vi "HTML_GetAllDepFromUsedPlugins.vi"(7 "Framwork Type":T1, 8 "Error In":errorcluster) -> (0 "Error Out":errorcluster, 1 "rel. Filepaths .js":path[](array[path]), 2 "rel. Filepaths .css":path[](array[path]))   [LabVIEW 2014]
uses:
  controls/StylingFrameworks_Enum.ctl
panel:
  # "Private:\nHTML_GetAllDepFromUsedPlugins.vi"
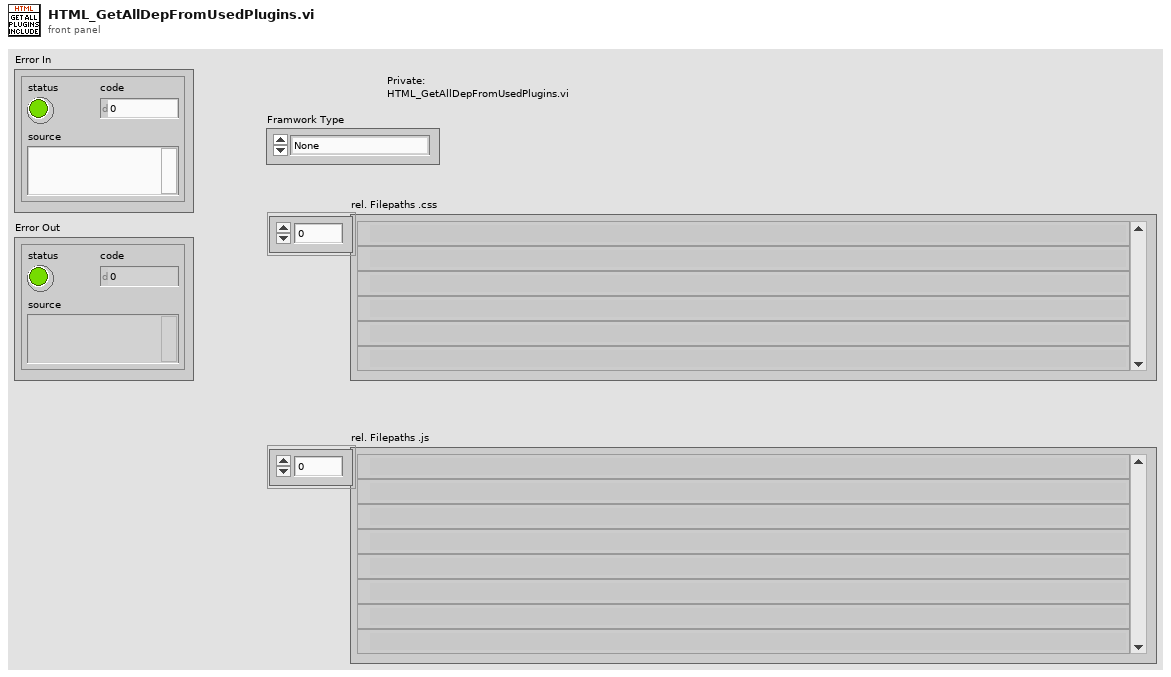
[diagram p1: front panel]
types:
  T1 = typedef "StylingFrameworks_Enum.ctl" = enum16{"None", "Bootstrap4", "Semantic-UI", "Custom"}
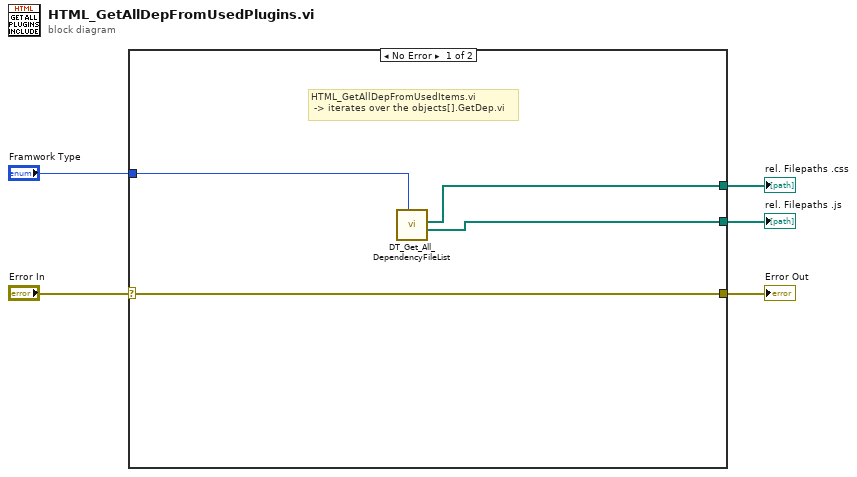
[diagram p0: block diagram]
diagram:
  n1 = case shown="No Error" "Error In" {
    selector: "Error In" -> [w9 w10]
    tunnel: [w9 w10] -> w4
    tunnel: "Framwork Type" -> [w8 _]
    tunnel: [w7 _] -> w2
    tunnel: [w6 _] -> w1
    frame No Error {
      # "HTML_GetAllDepFromUsedItems.vi\n -> iterates over the objects[].GetDep.vi"
      n2 = call "DT_Get_All_DependencyFileList.vi"("Framwork Type"=w8) -> ("rel. Filepaths .js"=w6:path[], "rel. Filepaths .css"=w7:path[])  [unwired: 9 in]
    }
    frame Error {
    }
  }
  "Error Out" <- w4
  "rel. Filepaths .css" <- w2
  "rel. Filepaths .js" <- w1
